vi "WMP Play File.vi"(8 "error in (no error)":errorcluster, 10 "File Path":path, 11 "Main Panel in":refnum<class "Main Panel.lvclass">) -> (0 "error out":errorcluster, 3 "Main Panel out":refnum<class "Main Panel.lvclass">)   [LabVIEW 2018, in "Main Panel.lvlib" / "Main Panel.lvclass"]
uses:
  Main Panel.lvclass
  Main Panel.lvclass/Main Panel.ctl
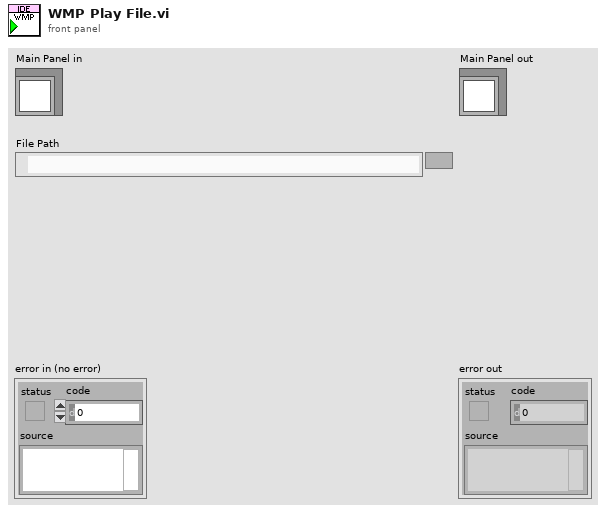
[diagram p1: front panel]
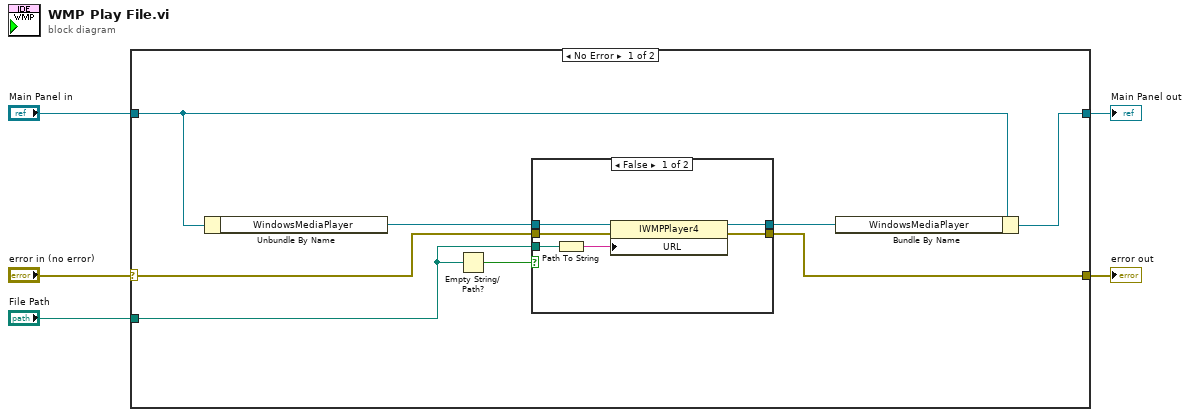
[diagram p0: block diagram]
diagram:
  n1 = case shown="No Error" "error in (no error)" {
    selector: "error in (no error)" -> [w6 w23]
    tunnel: [w8 w23] -> w4
    tunnel: [w12 w22] -> w2
    tunnel: "Main Panel in" -> [w13 w22]
    tunnel: "File Path" -> [w7 _]
    frame No Error {
      n2 = Unbundle By Name(w13) -> ("WindowsMediaPlayer"=w10:refnum<k7>)
      n3 = Empty String/Path?(string/path=w7) -> (empty?=w11:bool)
      n4 = case shown="False" w11 {
        tunnel: w7 -> [w15 _]
        tunnel: w10 -> [w19 w21]
        tunnel: [w18 w21] -> w9
        tunnel: [w17 w20] -> w8
        tunnel: w6 -> [w16 w20]
        frame False {
          n5 = Path To String(path=w15) -> (string=w14:string)
          n6 = property class="IWMPPlayer4"(reference=w19, error in=w16, "URL"=w14) -> (reference out=w18:refnum<k7>, error out=w17:errorcluster)
        }
        frame True {
          # "Invalid"
        }
      }
      n7 = Bundle By Name(cluster=w13, "WindowsMediaPlayer"=w9) -> (w12:refnum<class "Main Panel.lvclass">)
    }
    frame Error {
    }
  }
  "error out" <- w4
  "Main Panel out" <- w2
